vi "Open Audio File Read.vi"(8 "error in (no error)":errorcluster, 10 "Codec":string, 11 "Path":path) -> (0 "error out":errorcluster, 3 "Audio File Refnum":refnum<file>)   [LabVIEW 2020, in "G-Audio.lvlib"]
doc: "Opens an audio file and initializes the relevant decoder. If <b>codec</b> isn't specified, file extension determines the codec type.\n\nSupported codecs: flac, mp3, vorbis (ogg), and wav."
uses:
  G-Audio.lvlib
  Private/Get File Extension (Reentrant).vi
  <vilib>/Utility/error.llb/Error Cluster From Error Code.vi
  lib/g_audio_x86.dll
  lib/g_audio_x64.dll
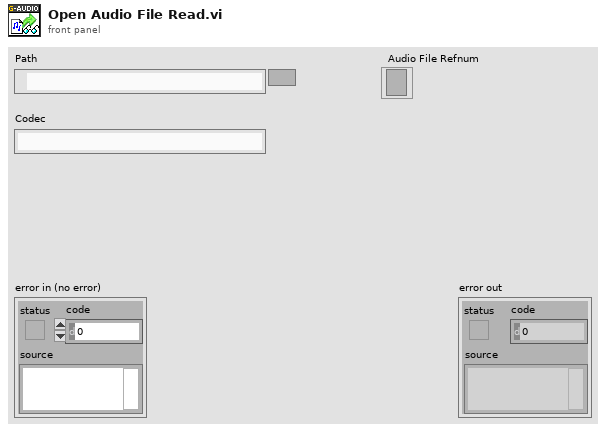
[diagram p1: front panel]
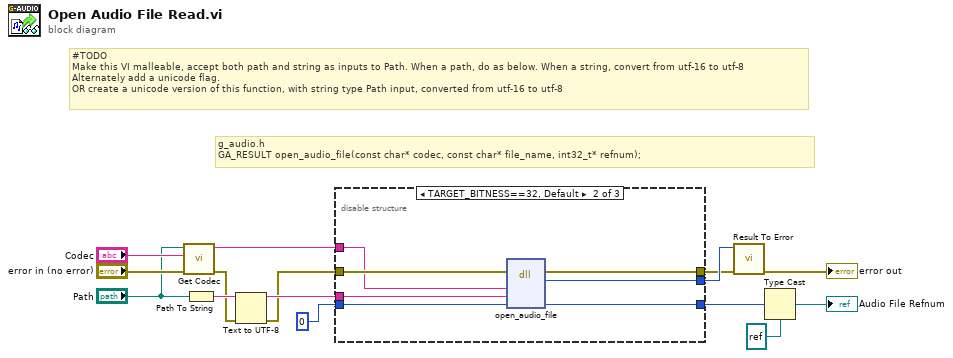
[diagram p0: block diagram]
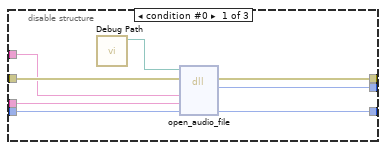
[diagram p2: hidden frame]
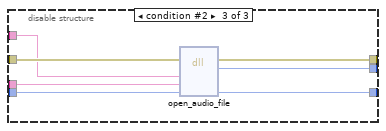
[diagram p3: hidden frame]
diagram:
  # "#TODO\nMake this VI malleable, accept both path and string as inputs to Path. When a path, do as below. When a string, convert from utf-16 to utf-8\nAlternately add a unicode flag.\nOR create a unicode version of this function, with string type Path input, converted from utf-16 to utf-8"
  # "g_audio.h\nGA_RESULT open_audio_file(const char* codec, const char* file_name, int32_t* refnum);"
  n1 = call "Get Codec.vi"("error in (no error)"="error in (no error)", "Codec In"="Codec", "Absolute Path"="Path") -> ("error out"=w3:errorcluster, "Codec Out"=w9:string)  [unwired: 7 in]
  n2 = Path To String(path="Path") -> (string=w5:string)
  n3 = Text to UTF-8(8:w3, 11:w5) -> (0:w2:errorcluster, 3:w4:string)  [unwired: 1 in]
  n4 = disable-structure shown="TARGET_BITNESS==32, Default" {
    disable-tunnel: w2 -> [w23 w30 w37]
    disable-tunnel: w4 -> [w21 w28 w35]
    disable-tunnel: [w22 w29 w36] -> w7
    disable-tunnel: 0 ("num_samples") -> [w19 w26 w33]
    disable-tunnel: w9 -> [w20 w27 w34]
    disable-tunnel: [w18 w25 w32] -> w13
    disable-tunnel: [w17 w24 w31] -> w8
    frame condition #0 {
      n5 = call "Debug Path.vi"() -> ("Debug Path"=w16:path)  [unwired: 11 in]
      n6 = dll-call lib="?" fn="open_audio_file"(path in=w16, error in=w23, "codec"=w20, "file_name"=w21, "refnum"=w19) -> (error out=w22:errorcluster, "result"=w17:i32, "refnum"=w18:i32)  [unwired: 3 in, 1 out]
    }
    frame condition #1 (active) {
      n7 = dll-call lib="C:/github/dataflowg/g-audio/src/LabVIEW/G-Audio/lib/g_audio_x86.*" fn="open_audio_file"(error in=w30, "codec"=w27, "file_name"=w28, "refnum"=w26) -> (error out=w29:errorcluster, "result"=w24:i32, "refnum"=w25:i32)  [unwired: 4 in, 1 out]
    }
    frame condition #2 {
      n8 = dll-call lib="C:/github/dataflowg/g-audio/src/LabVIEW/G-Audio/lib/g_audio_x64.*" fn="open_audio_file"(error in=w37, "codec"=w34, "file_name"=w35, "refnum"=w33) -> (error out=w36:errorcluster, "result"=w31:i32, "refnum"=w32:i32)  [unwired: 4 in, 1 out]
    }
  }
  n9 = call "Result To Error.vi"("error in (no error)"=w7, "Result Code"=w8) -> ("error out"=→"error out":errorcluster)  [unwired: 9 in]
  n10 = Type Cast(type=refnum<file> refnum ("Audio File Refnum"), x=w13) -> (*(type *) &x=→"Audio File Refnum":refnum<file>)
